vi "Run Function.vi"(0 "Message Popup in":refnum<class "Message Popup.lvclass">, 11 "error in (no error)":errorcluster) -> (4 "Message Popup out":refnum<class "Message Popup.lvclass">, 15 "error out":errorcluster)   [LabVIEW 2016, in "Message Popup.lvclass"]
uses:
  Message Popup.lvclass
  E:/Repository/LabVIEW Script Language/source code/LSL components/functions/functionsbase/functionbase.lvclass
  functionsbase/functionbase.lvclass/functionbase.ctl
  functionsbase/properties/Read Func Syntax.vi
  functionsbase/properties/Read Func Full String.vi
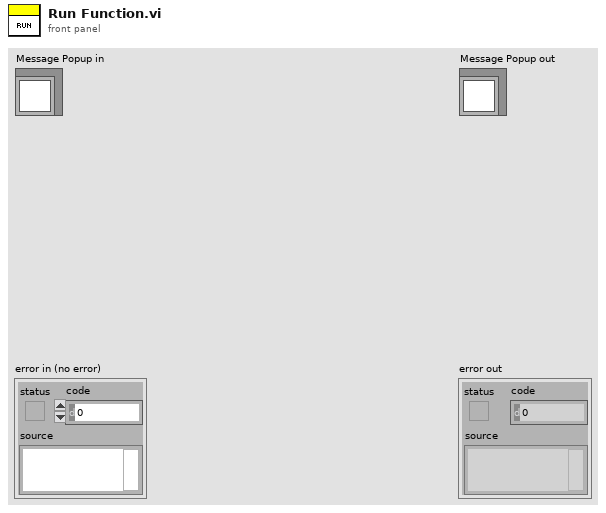
[diagram p1: front panel]
types:
  T1 = typedef "Syntax Format.ctl" = cluster{"Syntax":string, "Variable#":T2}
  T2 = typedef "Variable#.ctl" = enum16{"Zero", "One", "Two", "Three", "Four", "Five"}
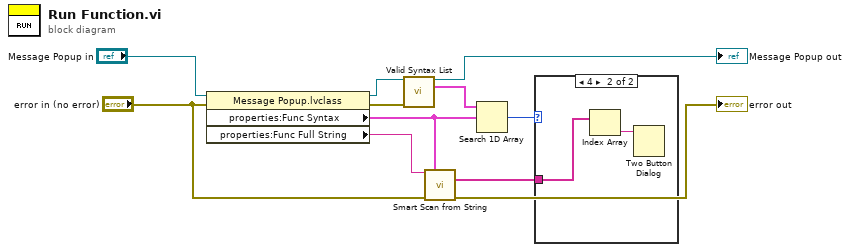
[diagram p0: block diagram]
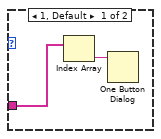
[diagram p2: hidden frame]
diagram:
  n1 = property class="Message Popup.lvclass"(reference="Message Popup in", error in="error in (no error)") -> (reference out=w2:refnum<class "Message Popup.lvclass">, error out=w6:errorcluster, "properties:Func Syntax"=w4:T1, "properties:Func Full String"=w10:string)
  n2 = call-dynamic "Valid Syntax List.vi"("Message Popup in"=w2, "error in (no error)"=w6) -> ("Message Popup out"=→"Message Popup out":refnum<class "Message Popup.lvclass">, "Syntax List"=w5:T1[])  [unwired: 11 in, 1 out]
  n3 = call "Smart Scan from String.vi"("initial string"=w10, "Syntax Format"=w4, "error in"="error in (no error)") -> ("Variables"=w7:string[], "error out"=→"error out":errorcluster)  [unwired: 10 in, 1 out]
  n4 = Search 1D Array(1D array=w5, element=w4) -> (index of element=w3:i32)  [unwired: 1 in]
  n5 = case shown="4" w3 {
    tunnel: w7 -> [w13 w15]
    frame 1, Default {
      n6 = Index Array(array=w13) -> (element=w12:string)  [unwired: 1 in]
      n7 = One Button Dialog(message=w12) -> ()  [unwired: 1 in, 1 out]
    }
    frame 4 {
      n8 = Index Array(array=w15) -> (element=w14:string)  [unwired: 1 in]
      n9 = Two Button Dialog(message=w14) -> ()  [unwired: 2 in, 1 out]
    }
  }
